vi "Add Decimal.vi"(8 "error in (no error)":errorcluster, 9 "Input Array":u16[](array[numeric])) -> (0 "error out":errorcluster, 1 "Output Array":u16[](array[numeric]))   [LabVIEW 2015]
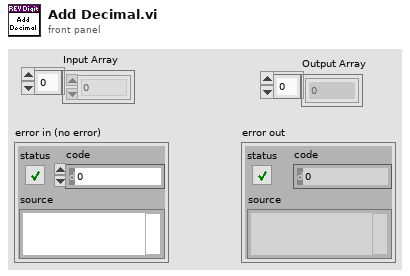
[diagram p1: front panel]
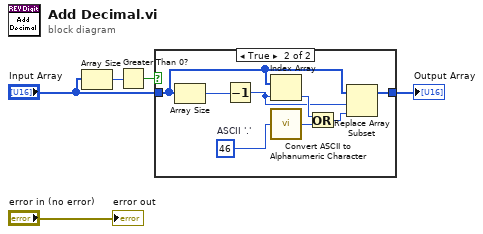
[diagram p0: block diagram]
diagram:
  n1 = Array Size(array="Input Array") -> (size(s)=w2:i32)
  n2 = Greater Than 0?(x=w2) -> (x > 0?=w1:bool)
  n3 = case shown="True" w1 {
    tunnel: "Input Array" -> [w6 w11]
    tunnel: [w6 w8] -> w4
    frame False {
    }
    frame True {
      w14 = u8 46  # ASCII '.'
      n4 = Array Size(array=w11) -> (size(s)=w10:i32)
      n5 = Decrement(x=w10) -> (x-1=w7:i32)
      n6 = Index Array(array=w11, index=w7) -> (element=w13:u16)
      n7 = call "Convert ASCII to Alphanumeric Character.vi"("ASCII Value"=w14) -> ("Alphanumeric Character Value"=w12:u16)
      n8 = Or(x=w13, y=w12) -> (x .or. y?=w9:u16)
      n9 = Replace Array Subset(array=w11, new element=w9, index=w7) -> (w8:u16[])
    }
  }
  "Output Array" <- w4
  "error out" <- "error in (no error)"
